vi "GetRGB.vi"(10 "sensors list":string[](array[string]), 11 "packet in":u8[](array[numeric])) -> (0 "blue":u16, 1 "green":u16, 2 "red":u16, 3 "light intensity":u16)   [LabVIEW 2018]
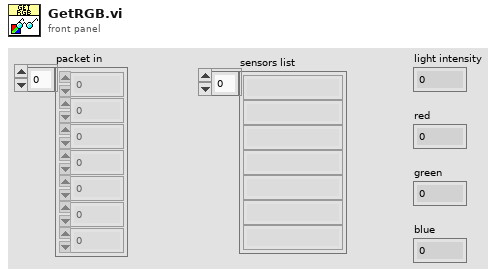
[diagram p1: front panel]
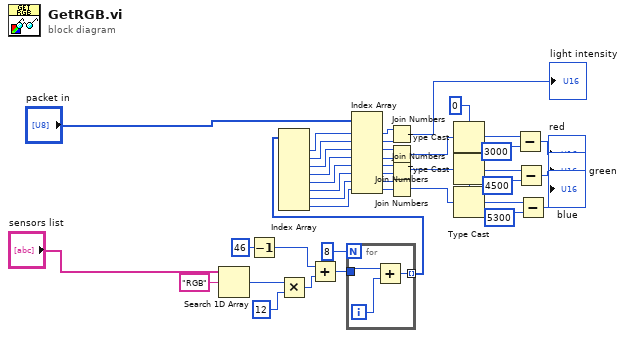
[diagram p0: block diagram]
diagram:
  w17 = u16 0 ("index")
  n1 = Search 1D Array(1D array="sensors list", element="RGB") -> (index of element=w14:i32)  [unwired: 1 in]
  n2 = Decrement(x=46) -> (x-1=w16:i32)
  n3 = Multiply(x=w14, y=12) -> (x*y=w15:i32)
  n4 = Add(x=w16, y=w15) -> (x+y=w9:i32)
  n5 = for {
    N: 8 -> [_]
    tunnel: w9 -> [w44]
    tunnel: [w43] -> w7 mode=indexing
    i -> [w42]
    n6 = Add(x=w44, y=w42) -> (x+y=w43:i32)
  }
  n7 = Index Array(array=w7) -> (element #1=w38:i32, element #2=w37:i32, element #3=w6:i32, element #4=w5:i32, element #5=w4:i32, element #6=w3:i32, element #7=w2:i32, element #8=w1:i32)  [unwired: 8 in]
  n8 = Index Array(array="packet in", index #1=w38, index #2=w37, index #3=w6, index #4=w5, index #5=w4, index #6=w3, index #7=w2, index #8=w1) -> (element #1=w40:u8, element #2=w39:u8, element #3=w19:u8, element #4=w20:u8, element #5=w21:u8, element #6=w22:u8, element #7=w23:u8, element #8=w24:u8)
  n9 = Join Numbers(hi=w40, lo=w39) -> ((hi.lo)=→"light intensity":u16)
  n10 = Join Numbers(hi=w19, lo=w20) -> ((hi.lo)=w25:u16)
  n11 = Join Numbers(hi=w22, lo=w21) -> ((hi.lo)=w26:u16)
  n12 = Join Numbers(hi=w24, lo=w23) -> ((hi.lo)=w27:u16)
  n13 = Type Cast(type=w17, x=w25) -> (*(type *) &x=w28:u16)
  n14 = Type Cast(type=w17, x=w26) -> (*(type *) &x=w34:u16)
  n15 = Type Cast(type=w17, x=w27) -> (*(type *) &x=w35:u16)
  n16 = Subtract(x=w28, y=u16 3000) -> (x-y=→"red":u16)
  n17 = Subtract(x=w34, y=u16 4500) -> (x-y=→"green":u16)
  n18 = Subtract(x=w35, y=u16 5300) -> (x-y=→"blue":u16)
